vi "Drona Path.vi"(0 "Control reference":refnum<vi>, 5 "Active VI reference":refnum<vi>, 11 "error in (no error)":errorcluster) -> (4 "Drona Path":string, 15 "error out":errorcluster)   [LabVIEW 2016, in "Drona Path obtn.lvlib"]
doc: "This VI is used to get the drona path of a control , with required inputs as Control reference and active VI reference"
uses:
  Drona Path obtn.lvlib
  Typedefs/Data container.ctl
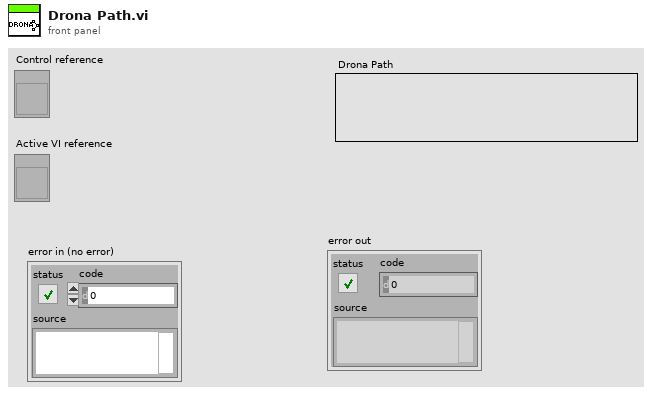
[diagram p1: front panel]
types:
  T1 = typedef "Drona Path obtn.lvlib/Data container.ctl" = cluster{"Subpanel TF":bool, "Path":string, "Subpanel ref":refnum<vi>}
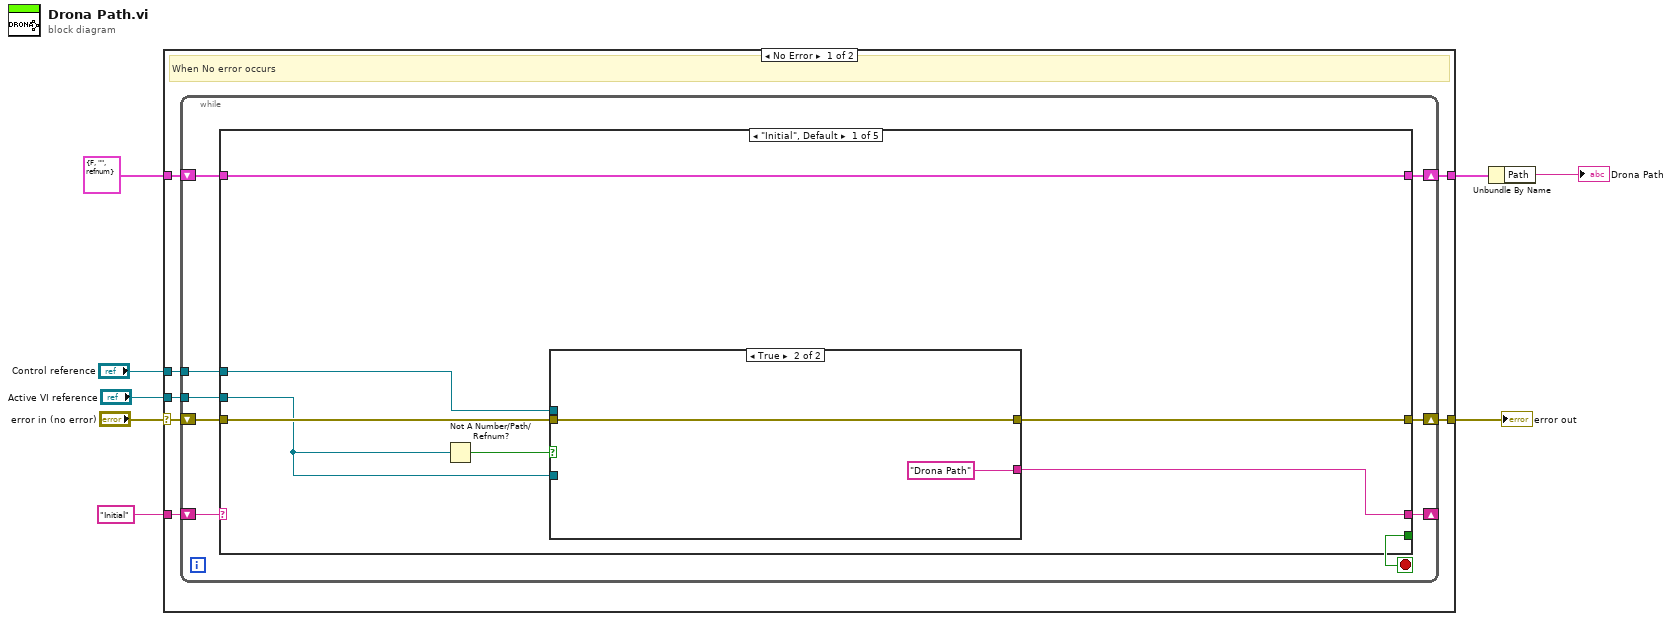
[diagram p0: block diagram]
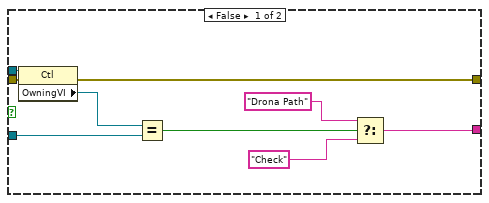
[diagram p2: hidden frame]
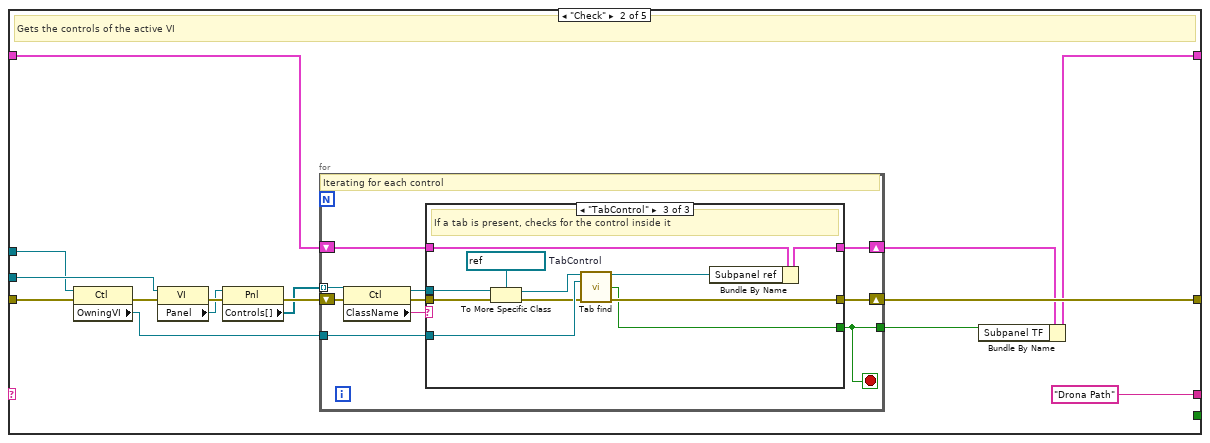
[diagram p3: hidden frame]
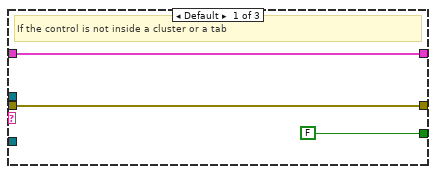
[diagram p4: hidden frame]
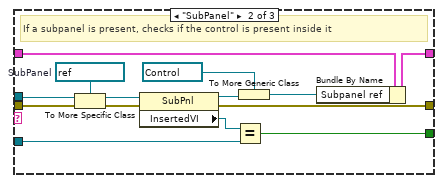
[diagram p5: hidden frame]
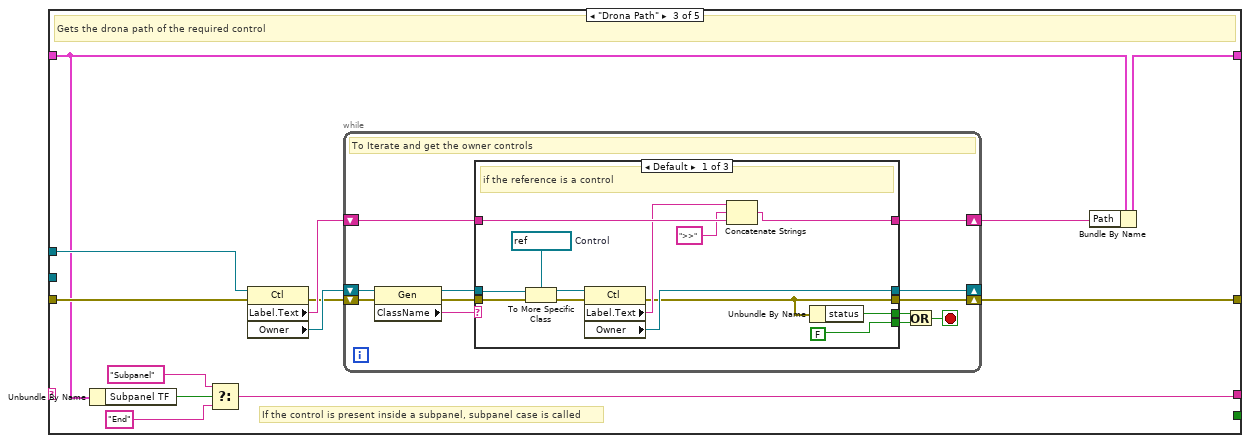
[diagram p6: hidden frame]
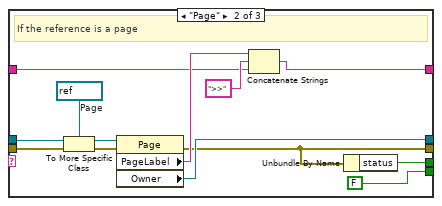
[diagram p7: hidden frame]
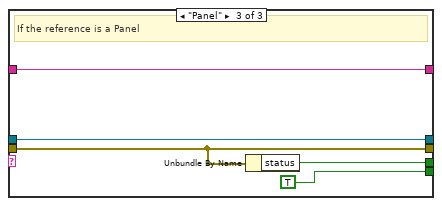
[diagram p8: hidden frame]
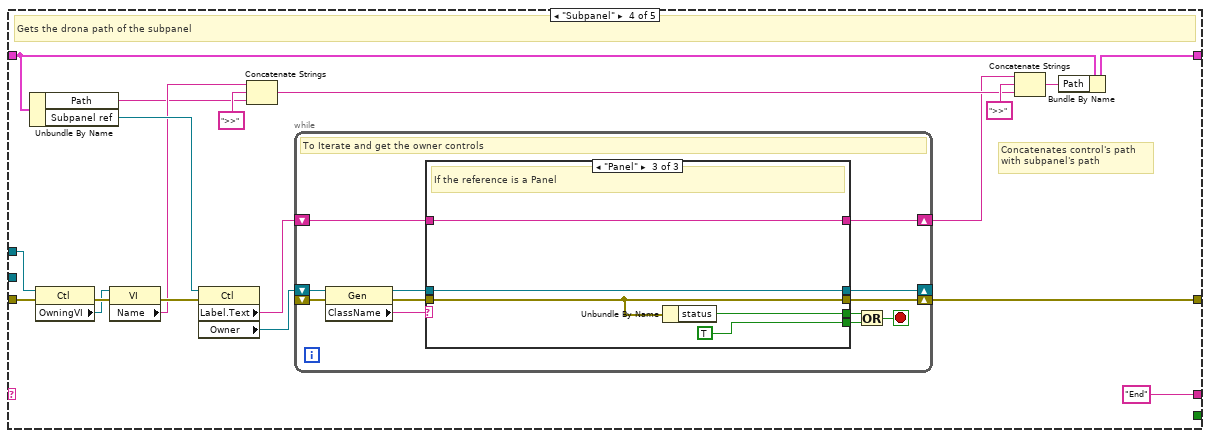
[diagram p9: hidden frame]
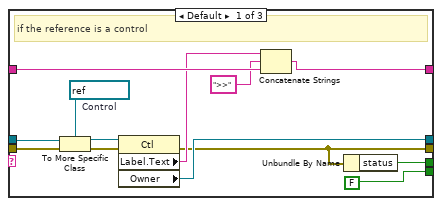
[diagram p10: hidden frame]
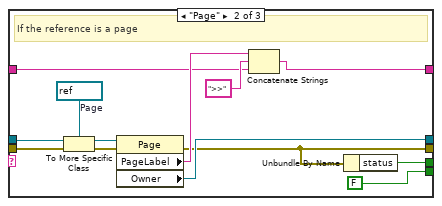
[diagram p11: hidden frame]
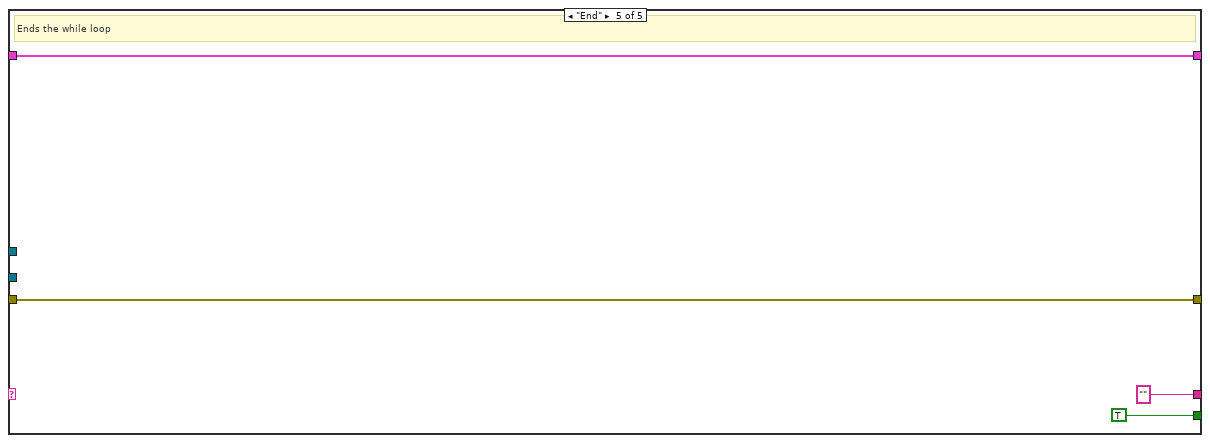
[diagram p12: hidden frame]
diagram:
  n1 = case shown="No Error" "error in (no error)" {
    selector: "error in (no error)" -> [w14 w219]
    tunnel: [w13 w219] -> w7
    tunnel: "Initial" -> [w15 _]
    tunnel: "Active VI reference" -> [w12 _]
    tunnel: "Control reference" -> [w11 _]
    tunnel: T1 {"Subpanel TF"=FALSE, "Path"="", "Subpanel ref"=refnum} -> [w10 w218]
    tunnel: [w9 w218] -> w2
    frame No Error {
      # "When No error occurs"
      n2 = while {
        tunnel: w12 -> [w21]
        tunnel: w11 -> [w20]
        shift-right: [w22] -> w13
        shift-left: w14 -> [w23]
        shift-right: [w18] -> w9
        shift-left: w10 -> [w19]
        shift-right: [w17] -> _
        shift-left: w15 -> [w24]
        stop <- w16 stop-if-true
        n3 = case shown="\"Initial\", Default" w24 {
          tunnel: w23 -> [w30 w57 w108 w169 w214]
          tunnel: [w28 w56 w107 w167 w214] -> w22
          tunnel: w21 -> [w25 w54 _ _ _]
          tunnel: w20 -> [w27 w49 w106 w164 _]
          tunnel: w19 -> [w31 w44 w105 w154 w215]
          tunnel: [w31 w47 w104 w153 w215] -> w18
          tunnel: [w29 "Drona Path" w96 "End" ("f") "" ("f")] -> w17
          tunnel: [_ _ _ _ TRUE] -> w16
          frame "Initial", Default {
            n4 = Not A Number/Path/Refnum?(number/path/refnum=w25) -> (NaN/Path/Refnum?=w26:bool)
            n5 = case shown="True" w26 {
              tunnel: w30 -> [w40 w42]
              tunnel: [w39 "Drona Path" ("f")] -> w29
              tunnel: [w36 w42] -> w28
              tunnel: w27 -> [w35 _]
              tunnel: w25 -> [w34 _]
              frame False {
                n6 = property class="Ctl"(reference=w35, error in=w40) -> (error out=w36:errorcluster, "OwningVI"=w33:refnum<vi>)  [unwired: 1 out]
                n7 = Equal?(x=w33, y=w34) -> (x = y?=w32:bool)
                n8 = Select(t="Drona Path" ("f"), s=w32, f="Check") -> (s? t:f=w39:string)
              }
              frame True {
              }
            }
          }
          frame "Check" {
            # "Gets the controls of the active VI"
            n9 = property class="Ctl"(reference=w49, error in=w57) -> (error out=w50:errorcluster, "OwningVI"=w48:refnum<vi>)  [unwired: 1 out]
            n10 = property class="VI"(reference=w54, error in=w50) -> (error out=w55:errorcluster, "Panel"=w52:refnum<vi>)  [unwired: 1 out]
            n11 = property class="Pnl"(reference=w52, error in=w55) -> (error out=w53:errorcluster, "Controls[]"=w51:refnum<vi>[])  [unwired: 1 out]
            n12 = for {
              shift-right: [w63] -> w56
              shift-left: w53 -> [w67]
              tunnel: w51 -> [w66] mode=indexing
              tunnel: w48 -> [w61]
              tunnel: [w58] -> w45
              shift-right: [w59] -> w43
              shift-left: w44 -> [w60]
              stop <- w58 stop-if-true
              # "Iterating for each control"
              n13 = property class="Ctl"(reference=w66, error in=w67) -> (reference out=w62:refnum<vi>, error out=w64:errorcluster, "ClassName"=w65:string)
              n14 = case shown="\"TabControl\"" w65 {
                tunnel: w64 -> [w70 w84 w95]
                tunnel: [w70 w76 w94] -> w63
                tunnel: w62 -> [_ w82 w87]
                tunnel: w61 -> [_ w78 w89]
                tunnel: [FALSE w77 w90] -> w58
                tunnel: w60 -> [w68 w75 w93]
                tunnel: [w68 w74 w92] -> w59
                frame Default {
                  # "If the control is not inside a cluster or a tab"
                }
                frame "SubPanel" {
                  w80 = refnum<vi> refnum  # SubPanel
                  # "If a subpanel is present, checks if the control is present inside it"
                  n15 = To More Specific Class(target class=w80, reference=w82, error in=w84) -> (specific class reference=w81:refnum<vi>, error out=w83:errorcluster)
                  n16 = property class="SubPnl"(reference=w81, error in=w83) -> (reference out=w73:refnum<vi>, error out=w76:errorcluster, "InsertedVI"=w79:refnum<vi>)
                  n17 = Equal?(x=w79, y=w78) -> (x = y?=w77:bool)
                  n18 = To More Generic Class(target class=refnum<vi> refnum ("Ctl Refnum"), reference=w73) -> (generic class reference=w71:refnum<vi>)
                  n19 = Bundle By Name(cluster=w75, "Subpanel ref"=w71) -> (w74:T1)
                }
                frame "TabControl" {
                  w85 = refnum<vi> refnum  # TabControl
                  # "If a tab is present, checks for the control inside it"
                  n20 = To More Specific Class(target class=w85, reference=w87, error in=w95) -> (specific class reference=w86:refnum<vi>, error out=w88:errorcluster)
                  n21 = call "Tab find.vi"("TabCtl Refnum"=w86, "VI Refnum"=w89, "error in (no error)"=w88) -> ("SP ref out"=w91:refnum<vi>, "Boolean"=w90:bool, "error out"=w94:errorcluster)  [unwired: 10 in]
                  n22 = Bundle By Name(cluster=w93, "Subpanel ref"=w91) -> (w92:T1)
                }
              }
            }
            n23 = Bundle By Name(cluster=w43, "Subpanel TF"=w45) -> (w47:T1)
          }
          frame "Drona Path" {
            # "If the control is present inside a subpanel, subpanel case is called"
            # "Gets the drona path of the required control"
            n24 = Unbundle By Name(w105) -> ("Subpanel TF"=w99:bool)
            n25 = Select(t="Subpanel", s=w99, f="End") -> (s? t:f=w96:string)
            n26 = property class="Ctl"(reference=w106, error in=w108) -> (error out=w100:errorcluster, "Label.Text"=w102:string, "Owner"=w101:refnum<vi>)  [unwired: 1 out]
            n27 = while {
              shift-right: [w115] -> w107
              shift-left: w100 -> [w120]
              shift-right: [w113] -> w103
              shift-left: w102 -> [w114]
              shift-right: [w112] -> _
              shift-left: w101 -> [w119]
              stop <- w111 stop-if-true
              # "To Iterate and get the owner controls"
              n28 = property class="Gen"(reference=w119, error in=w120) -> (reference out=w117:refnum<vi>, error out=w116:errorcluster, "ClassName"=w118:string)
              n29 = case shown="Default" w118 {
                tunnel: w117 -> [w131 w144 w149]
                tunnel: w116 -> [w133 w146 w148]
                tunnel: [w123 w136 w148] -> w115
                tunnel: [FALSE FALSE TRUE] -> w110
                tunnel: w114 -> [w127 w139 w150]
                tunnel: [w125 w138 w150] -> w113
                tunnel: [w128 w137 w149] -> w112
                tunnel: [w122 w135 w147] -> w109
                frame Default {
                  w130 = refnum<vi> refnum  # Control
                  # "if the reference is a control"
                  n30 = To More Specific Class(target class=w130, reference=w131, error in=w133) -> (specific class reference=w129:refnum<vi>, error out=w132:errorcluster)
                  n31 = property class="Ctl"(reference=w129, error in=w132) -> (error out=w123:errorcluster, "Label.Text"=w126:string, "Owner"=w128:refnum<vi>)  [unwired: 1 out]
                  n32 = Concatenate Strings(w126, ">>" ("string"), w127) -> (w125:string)
                  n33 = Unbundle By Name(w123) -> ("status"=w122:bool)
                }
                frame "Page" {
                  w143 = refnum<vi> refnum  # Page
                  # "If the reference is a page"
                  n34 = To More Specific Class(target class=w143, reference=w144, error in=w146) -> (specific class reference=w142:refnum<vi>, error out=w145:errorcluster)
                  n35 = property class="Page"(reference=w142, error in=w145) -> (error out=w136:errorcluster, "PageLabel"=w140:string, "Owner"=w137:refnum<vi>)  [unwired: 1 out]
                  n36 = Concatenate Strings(w140, ">>" ("string"), w139) -> (w138:string)
                  n37 = Unbundle By Name(w136) -> ("status"=w135:bool)
                }
                frame "Panel" {
                  # "If the reference is a Panel"
                  n38 = Unbundle By Name(w148) -> ("status"=w147:bool)
                }
              }
              n39 = Or(x=w109, y=w110) -> (x .or. y?=w111:bool)
            }
            n40 = Bundle By Name(cluster=w105, "Path"=w103) -> (w104:T1)
          }
          frame "Subpanel" {
            # "Concatenates control's path \nwith subpanel's path"
            # "Gets the drona path of the subpanel"
            n41 = Unbundle By Name(w154) -> ("Path"=w159:string, "Subpanel ref"=w166:refnum<vi>)
            n42 = property class="Ctl"(reference=w164, error in=w169) -> (error out=w165:errorcluster, "OwningVI"=w162:refnum<vi>)  [unwired: 1 out]
            n43 = property class="VI"(reference=w162, error in=w165) -> (error out=w163:errorcluster, "Name"=w161:string)  [unwired: 1 out]
            n44 = property class="Ctl"(reference=w166, error in=w163) -> ("Label.Text"=w170:string, "Owner"=w168:refnum<vi>)  [unwired: 2 out]
            n45 = Concatenate Strings(w161, ">>" ("string"), w159) -> (w157:string)
            n46 = while {
              shift-right: [w177] -> w167
              shift-left: _ -> [w182]
              shift-right: [w175] -> w156
              shift-left: w170 -> [w176]
              shift-right: [w174] -> _
              shift-left: w168 -> [w181]
              stop <- w173 stop-if-true
              # "To Iterate and get the owner controls"
              n47 = property class="Gen"(reference=w181, error in=w182) -> (reference out=w179:refnum<vi>, error out=w178:errorcluster, "ClassName"=w180:string)
              n48 = case shown="\"Panel\"" w180 {
                tunnel: w179 -> [w193 w206 w211]
                tunnel: w178 -> [w195 w208 w210]
                tunnel: [w185 w198 w210] -> w177
                tunnel: [FALSE FALSE TRUE] -> w172
                tunnel: w176 -> [w189 w201 w212]
                tunnel: [w187 w200 w212] -> w175
                tunnel: [w190 w199 w211] -> w174
                tunnel: [w184 w197 w209] -> w171
                frame Default {
                  w192 = refnum<vi> refnum  # Control
                  # "if the reference is a control"
                  n49 = To More Specific Class(target class=w192, reference=w193, error in=w195) -> (specific class reference=w191:refnum<vi>, error out=w194:errorcluster)
                  n50 = property class="Ctl"(reference=w191, error in=w194) -> (error out=w185:errorcluster, "Label.Text"=w188:string, "Owner"=w190:refnum<vi>)  [unwired: 1 out]
                  n51 = Concatenate Strings(w188, ">>" ("string"), w189) -> (w187:string)
                  n52 = Unbundle By Name(w185) -> ("status"=w184:bool)
                }
                frame "Page" {
                  w205 = refnum<vi> refnum  # Page
                  # "If the reference is a page"
                  n53 = To More Specific Class(target class=w205, reference=w206, error in=w208) -> (specific class reference=w204:refnum<vi>, error out=w207:errorcluster)
                  n54 = property class="Page"(reference=w204, error in=w207) -> (error out=w198:errorcluster, "PageLabel"=w202:string, "Owner"=w199:refnum<vi>)  [unwired: 1 out]
                  n55 = Concatenate Strings(w202, ">>" ("string"), w201) -> (w200:string)
                  n56 = Unbundle By Name(w198) -> ("status"=w197:bool)
                }
                frame "Panel" {
                  # "If the reference is a Panel"
                  n57 = Unbundle By Name(w210) -> ("status"=w209:bool)
                }
              }
              n58 = Or(x=w171, y=w172) -> (x .or. y?=w173:bool)
            }
            n59 = Concatenate Strings(w156, ">>" ("string"), w157) -> (w155:string)
            n60 = Bundle By Name(cluster=w154, "Path"=w155) -> (w153:T1)
          }
          frame "End" {
            # "Ends the while loop"
          }
        }
      }
    }
    frame Error {
    }
  }
  "error out" <- w7
  n61 = Unbundle By Name(w2) -> ("Path"=→"Drona Path":string)
